vi "Add Common Data.vi"(8 "error in (no error)":errorcluster, 9 "TestStand Result":T1, 10 "Empty Row":string[](array[string]), 11 "Result Handler":refnum<class "TestStand Result Handler.lvclass">) -> (0 "error out":errorcluster, 2 "Array":string[](array[string]), 3 "Result Handler 2":refnum<class "TestStand Result Handler.lvclass">)   [LabVIEW 2020, in "Astemes_CSVReportPlugin.lvlib" / "TestStand Result Handler.lvclass"]
uses:
  TestStand Result Handler.lvclass
  TestStand Result.ctl
  Columns.ctl
  TestStand Result Handler.lvclass/TestStand Result Handler.ctl
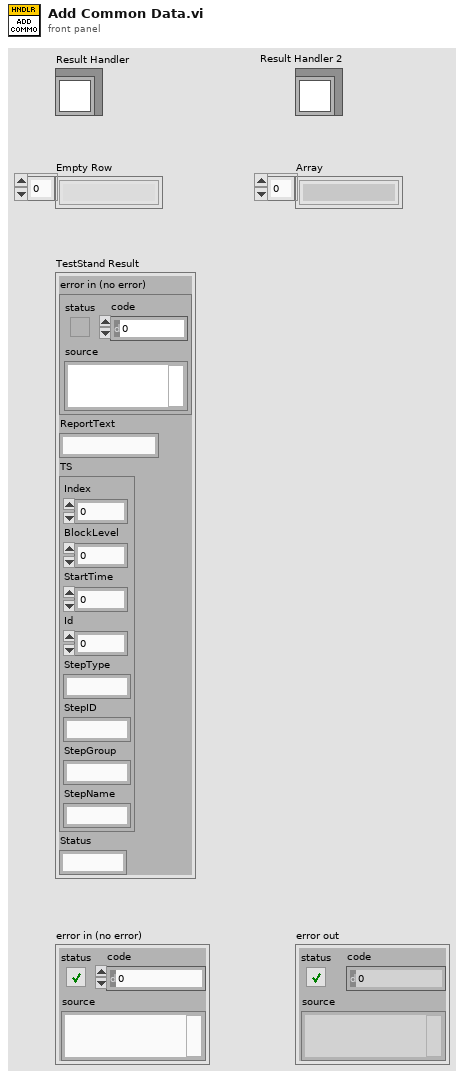
[diagram p1: front panel]
types:
  T1 = typedef "Astemes_CSVReportPlugin.lvlib/TestStand Result Handler.lvclass/TestStand Result.ctl" = cluster{"error in (no error)":errorcluster, "ReportText":string, "TS":cluster{"Index":i32, "BlockLevel":i32, "StartTime":dbl, "Id":i32, "StepType":string, "StepID":string, "StepGroup":string, "StepName":string}, "Status":string}
  T2 = typedef "Astemes_CSVReportPlugin.lvlib/TestStand Result Handler.lvclass/Columns.ctl" = enum16{"StepName", "Result", "LowerLimit", "ComparisonTypeLow", "Measurement", "ComparisonTypeHigh", "UpperLimit", "ReportText", "StepType"}
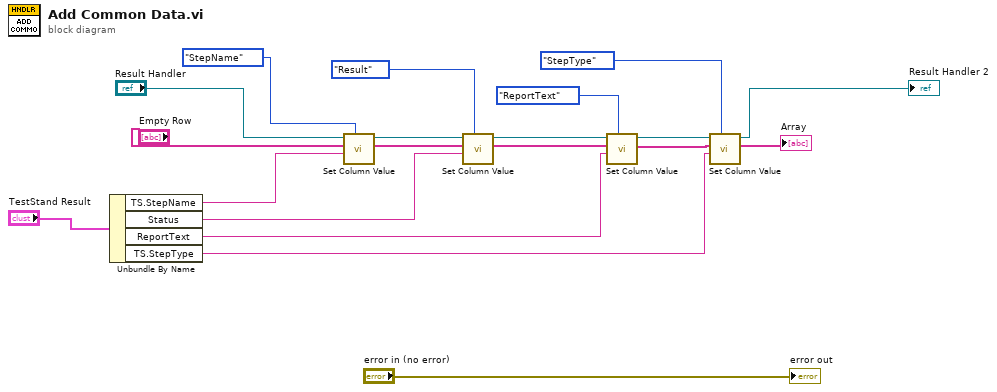
[diagram p0: block diagram]
diagram:
  n1 = Unbundle By Name("TestStand Result") -> ("TS.StepName"=w18:string, "Status"=w19:string, "ReportText"=w20:string, "TS.StepType"=w14:string)
  n2 = call "Set Column Value.vi"("Column"=Columns."StepName", "Value"=w18, "Row In"="Empty Row", "Result Handler"="Result Handler") -> ("Row Out"=w5:string[], "Result Handler Out"=w16:refnum<class "TestStand Result Handler.lvclass">)  [unwired: 6 in]
  n3 = call "Set Column Value.vi"("Column"=Columns."Result", "Value"=w19, "Row In"=w5, "Result Handler"=w16) -> ("Row Out"=w6:string[], "Result Handler Out"=w8:refnum<class "TestStand Result Handler.lvclass">)  [unwired: 6 in]
  n4 = call "Set Column Value.vi"("Column"=Columns."ReportText", "Value"=w20, "Row In"=w6, "Result Handler"=w8) -> ("Row Out"=w4:string[], "Result Handler Out"=w15:refnum<class "TestStand Result Handler.lvclass">)  [unwired: 6 in]
  n5 = call "Set Column Value.vi"("Column"=Columns."StepType", "Value"=w14, "Row In"=w4, "Result Handler"=w15) -> ("Row Out"=→"Array":string[], "Result Handler Out"=→"Result Handler 2":refnum<class "TestStand Result Handler.lvclass">)  [unwired: 6 in]
  "error out" <- "error in (no error)"
